vi "S7_1200.vi"() -> ()   [LabVIEW 2024]
uses:
  <vilib>/OPCUA/NI OPC UA Client.lvlib
panel:
  out "EV2.3":T1
  out "EV2.2":T1
  out "EV2.1":T1
  out "EV1.3":T1
  out "EV1.2":T1
  out "EV1.1":T1
  out "VALUES READ":map{string, i32}(c390)
  out "Coils read":map{string, bool}(c390)
  in  "stop":bool
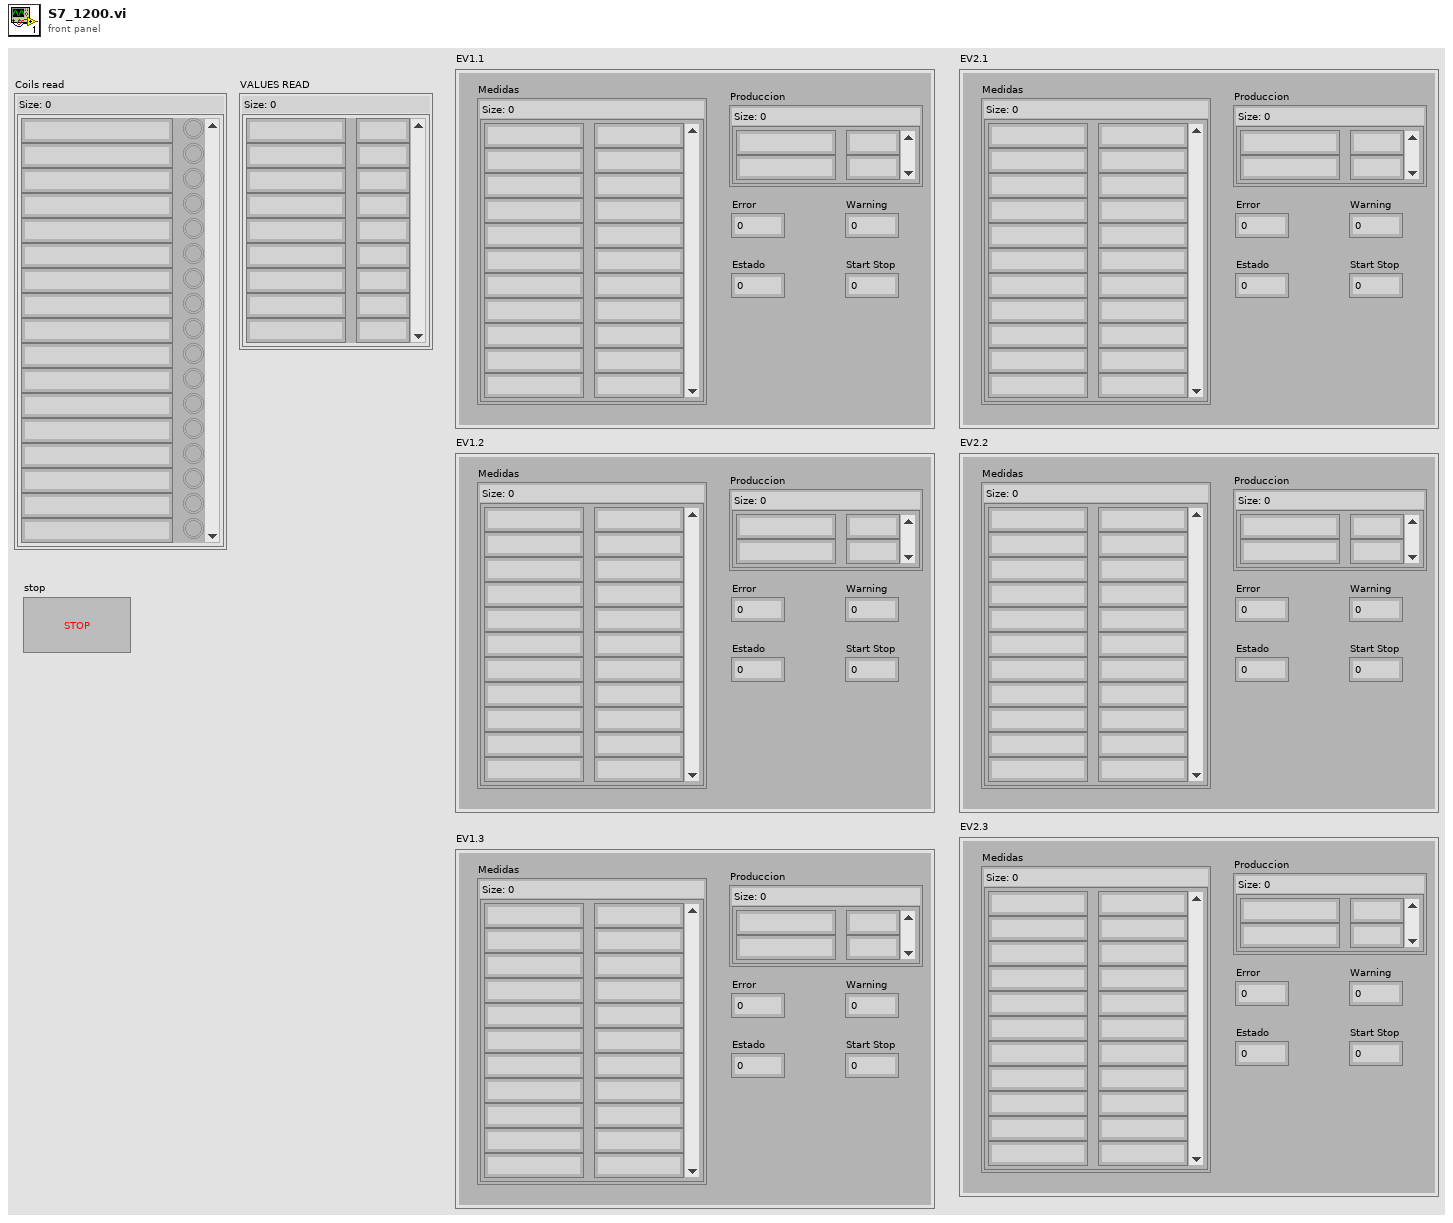
[diagram p1: front panel]
types:
  T1 = cluster{"Medidas":map{string, dbl}, "Produccion":map{string, dbl}, "Warning":u16, "Error":u16, "Estado":u16, "Start Stop":u16}
  T2 = cluster{"message mode":enum16{"None", "Sign", "Sign and Encrypt"}, "security":enum16{"Basic256", "Basic128Rsa15"}}
  T3 = typedef "OPC UA Client Refnum.ctl" = refnum<k21>
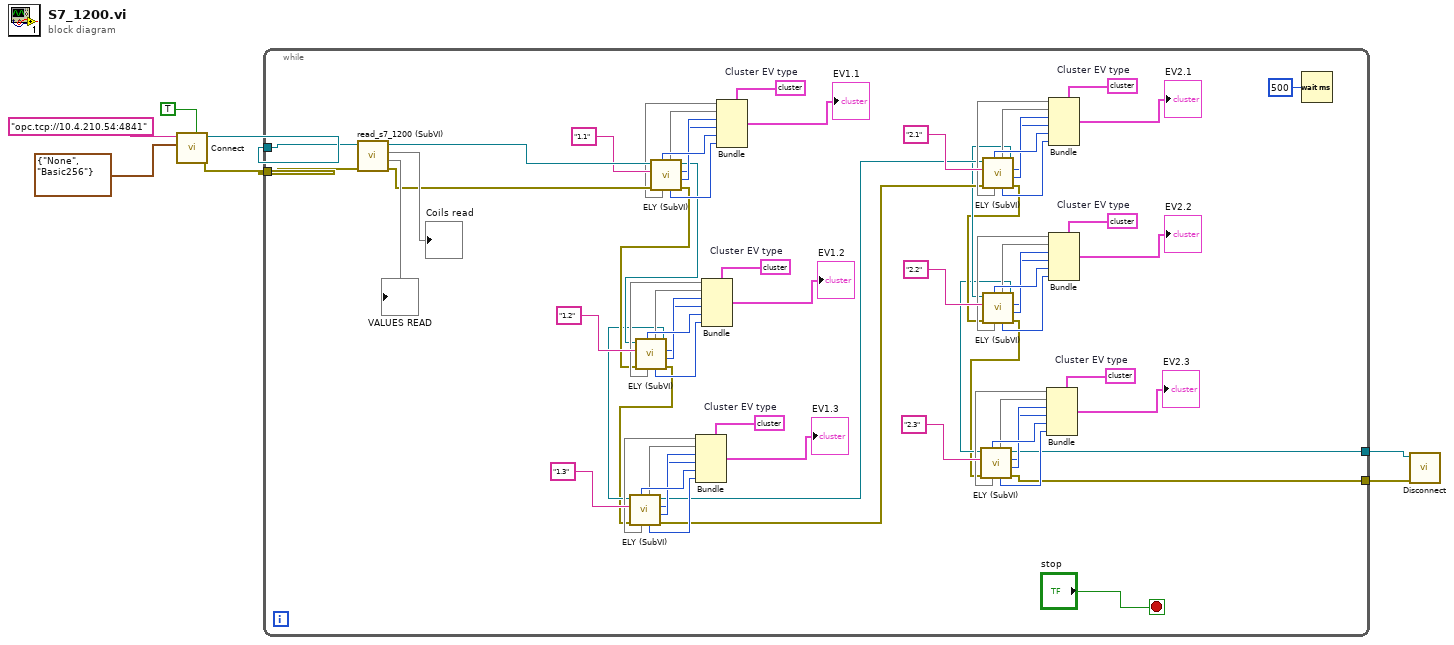
[diagram p0: block diagram]
diagram:
  n1 = call <vilib>:"Connect.vi"("trust any server (F)"=TRUE, "security policy"=T2 {"message mode"=enum."None", "security"=enum."Basic256"}, "server endpoint URL"="opc.tcp://10.4.210.54:4841") -> ("error out"=w3:errorcluster, "OPC UA client refnum out"=w4:T3)  [unwired: 6 in, 1 out]
  n2 = while {
    tunnel: w4 -> [w81]
    tunnel: w3 -> [w80]
    tunnel: [w9] -> w2
    tunnel: [w8] -> w1
    stop <- "stop" stop-if-true
    w23 = T1 {"Medidas"={"Medidas[10]"=13.862751007080078, "Medidas[11]"=14.109219551086426, "Medidas[1]"=0.0, "Medidas[2]"=4080.0, "Medidas[3]"=0.0, "Medidas[4]"=4.289261817932129, "Medidas[5]"=0.18084581196308136, "Medidas[6]"=5.004517078399658, "Medidas[7]"=-0.1899999976158142, "Medidas[8]"=-0.06411409378051758, "Medidas[9]"=1.6946747303009033}, "Produccion"={"Produccion[1]"=70208.90625, "Produccion[2]"=0.0}, "Warning"=0, "Error"=0, "Estado"=3, "Start Stop"=0}  # Cluster EV type
    w32 = T1 {"Medidas"={"Medidas[10]"=13.862751007080078, "Medidas[11]"=14.109219551086426, "Medidas[1]"=0.0, "Medidas[2]"=4080.0, "Medidas[3]"=0.0, "Medidas[4]"=4.289261817932129, "Medidas[5]"=0.18084581196308136, "Medidas[6]"=5.004517078399658, "Medidas[7]"=-0.1899999976158142, "Medidas[8]"=-0.06411409378051758, "Medidas[9]"=1.6946747303009033}, "Produccion"={"Produccion[1]"=70208.90625, "Produccion[2]"=0.0}, "Warning"=0, "Error"=0, "Estado"=3, "Start Stop"=0}  # Cluster EV type
    w41 = T1 {"Medidas"={"Medidas[10]"=13.862751007080078, "Medidas[11]"=14.109219551086426, "Medidas[1]"=0.0, "Medidas[2]"=4080.0, "Medidas[3]"=0.0, "Medidas[4]"=4.289261817932129, "Medidas[5]"=0.18084581196308136, "Medidas[6]"=5.004517078399658, "Medidas[7]"=-0.1899999976158142, "Medidas[8]"=-0.06411409378051758, "Medidas[9]"=1.6946747303009033}, "Produccion"={"Produccion[1]"=70208.90625, "Produccion[2]"=0.0}, "Warning"=0, "Error"=0, "Estado"=3, "Start Stop"=0}  # Cluster EV type
    w54 = T1 {"Medidas"={"Medidas[10]"=13.862751007080078, "Medidas[11]"=14.109219551086426, "Medidas[1]"=0.0, "Medidas[2]"=4080.0, "Medidas[3]"=0.0, "Medidas[4]"=4.289261817932129, "Medidas[5]"=0.18084581196308136, "Medidas[6]"=5.004517078399658, "Medidas[7]"=-0.1899999976158142, "Medidas[8]"=-0.06411409378051758, "Medidas[9]"=1.6946747303009033}, "Produccion"={"Produccion[1]"=70208.90625, "Produccion[2]"=0.0}, "Warning"=0, "Error"=0, "Estado"=3, "Start Stop"=0}  # Cluster EV type
    w63 = T1 {"Medidas"={"Medidas[10]"=13.862751007080078, "Medidas[11]"=14.109219551086426, "Medidas[1]"=0.0, "Medidas[2]"=4080.0, "Medidas[3]"=0.0, "Medidas[4]"=4.289261817932129, "Medidas[5]"=0.18084581196308136, "Medidas[6]"=5.004517078399658, "Medidas[7]"=-0.1899999976158142, "Medidas[8]"=-0.06411409378051758, "Medidas[9]"=1.6946747303009033}, "Produccion"={"Produccion[1]"=70208.90625, "Produccion[2]"=0.0}, "Warning"=0, "Error"=0, "Estado"=3, "Start Stop"=0}  # Cluster EV type
    w72 = T1 {"Medidas"={"Medidas[10]"=13.862751007080078, "Medidas[11]"=14.109219551086426, "Medidas[1]"=0.0, "Medidas[2]"=4080.0, "Medidas[3]"=0.0, "Medidas[4]"=4.289261817932129, "Medidas[5]"=0.18084581196308136, "Medidas[6]"=5.004517078399658, "Medidas[7]"=-0.1899999976158142, "Medidas[8]"=-0.06411409378051758, "Medidas[9]"=1.6946747303009033}, "Produccion"={"Produccion[1]"=70208.90625, "Produccion[2]"=0.0}, "Warning"=0, "Error"=0, "Estado"=3, "Start Stop"=0}  # Cluster EV type
    n3 = call "read_s7_1200 (SubVI).vi"("error in (no error)"=w80, "Refnum in"=w81) -> ("error out"=w74:errorcluster, "VALUES READ"=→"VALUES READ":map{string, i32}, "Coils read"=→"Coils read":map{string, bool}, "Refnum out"=w75:T3)  [unwired: 6 in]
    n4 = call "ELY (SubVI).vi"("error in (no error)"=w74, "Electrolizador"="1.1", "Refnum in"=w75) -> ("error out"=w45:errorcluster, "Warning"=w68:u16, "Error"=w67:u16, "Refnum out"=w46:T3, "StartStop"=w69:u16, "Produccion"=w66:map{string, dbl}, "Medidas"=w65:map{string, dbl}, "Estado"=w70:u16)  [unwired: 1 in]
    n5 = call "ELY (SubVI).vi"("error in (no error)"=w45, "Electrolizador"="1.2", "Refnum in"=w46) -> ("error out"=w43:errorcluster, "Warning"=w59:u16, "Error"=w58:u16, "Refnum out"=w44:T3, "StartStop"=w60:u16, "Produccion"=w57:map{string, dbl}, "Medidas"=w56:map{string, dbl}, "Estado"=w61:u16)  [unwired: 1 in]
    n6 = call "ELY (SubVI).vi"("error in (no error)"=w43, "Electrolizador"="1.3", "Refnum in"=w44) -> ("error out"=w14:errorcluster, "Warning"=w50:u16, "Error"=w49:u16, "Refnum out"=w15:T3, "StartStop"=w51:u16, "Produccion"=w48:map{string, dbl}, "Medidas"=w47:map{string, dbl}, "Estado"=w52:u16)  [unwired: 1 in]
    n7 = Bundle(cluster=w54, "Medidas"=w47, "Produccion"=w48, "Warning"=w50, "Error"=w49, "Estado"=w52, "Start Stop"=w51) -> (→"EV1.3":T1)
    n8 = Bundle(cluster=w63, "Medidas"=w56, "Produccion"=w57, "Warning"=w59, "Error"=w58, "Estado"=w61, "Start Stop"=w60) -> (→"EV1.2":T1)
    n9 = Bundle(cluster=w72, "Medidas"=w65, "Produccion"=w66, "Warning"=w68, "Error"=w67, "Estado"=w70, "Start Stop"=w69) -> (→"EV1.1":T1)
    n10 = call "ELY (SubVI).vi"("error in (no error)"=w14, "Electrolizador"="2.1", "Refnum in"=w15) -> ("error out"=w12:errorcluster, "Warning"=w37:u16, "Error"=w36:u16, "Refnum out"=w13:T3, "StartStop"=w38:u16, "Produccion"=w35:map{string, dbl}, "Medidas"=w34:map{string, dbl}, "Estado"=w39:u16)  [unwired: 1 in]
    n11 = call "ELY (SubVI).vi"("error in (no error)"=w12, "Electrolizador"="2.2", "Refnum in"=w13) -> ("error out"=w10:errorcluster, "Warning"=w28:u16, "Error"=w27:u16, "Refnum out"=w11:T3, "StartStop"=w29:u16, "Produccion"=w26:map{string, dbl}, "Medidas"=w25:map{string, dbl}, "Estado"=w30:u16)  [unwired: 1 in]
    n12 = call "ELY (SubVI).vi"("error in (no error)"=w10, "Electrolizador"="2.3", "Refnum in"=w11) -> ("error out"=w8:errorcluster, "Warning"=w19:u16, "Error"=w18:u16, "Refnum out"=w9:T3, "StartStop"=w20:u16, "Produccion"=w17:map{string, dbl}, "Medidas"=w16:map{string, dbl}, "Estado"=w21:u16)  [unwired: 1 in]
    n13 = Bundle(cluster=w23, "Medidas"=w16, "Produccion"=w17, "Warning"=w19, "Error"=w18, "Estado"=w21, "Start Stop"=w20) -> (→"EV2.3":T1)
    n14 = Bundle(cluster=w41, "Medidas"=w34, "Produccion"=w35, "Warning"=w37, "Error"=w36, "Estado"=w39, "Start Stop"=w38) -> (→"EV2.1":T1)
    n15 = Bundle(cluster=w32, "Medidas"=w25, "Produccion"=w26, "Warning"=w28, "Error"=w27, "Estado"=w30, "Start Stop"=w29) -> (→"EV2.2":T1)
    n16 = Wait (ms)(milliseconds to wait=u32 500) -> ()  [unwired: 1 out]
  }
  n17 = call <vilib>:"Disconnect.vi"("error in (no error)"=w1, "OPC UA client refnum in"=w2) -> ()  [unwired: 9 in, 1 out]
